vi "Environment Step Type - Configure.vi"(9 "Value Expression In":string, 10 "Environment Setting":T1, 11 "Sequence Context In":refnum<k7>) -> (0 "error out":errorcluster, 1 "Setting name":string, 2 "Value Expression Out":string, 3 "Setting out":T1)   [LabVIEW 2013]
uses:
  <instrlib>/Driver Simulation/Fixture/EnvironmentSettings.ctl
  <vilib>/addons/TestStand/_TSUtility.llb/TestStand - Start Modal Dialog (Sequence Context).vi
  <vilib>/addons/TestStand/_TSUtility.llb/TestStand - End Modal Dialog (Sequence Context).vi
  <instrlib>/Driver Simulation/Fixture.lvlib
panel:
  in  "Cancel":bool
  in  "Value":refnum<k7>(container)
  in  "OK":bool
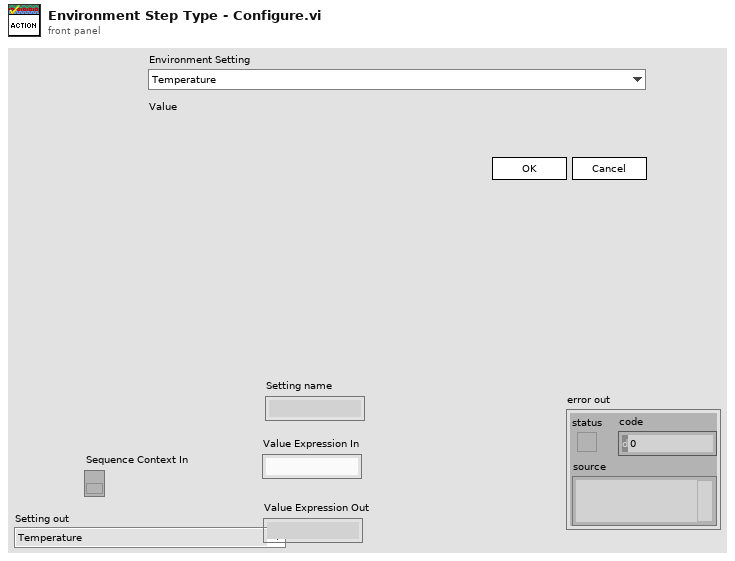
[diagram p1: front panel]
types:
  T1 = typedef "Driver Simulation.lvlib/Fixture.lvlib/EnvironmentSettings.ctl" = enum16{"Temperature", "Light Intensity"}
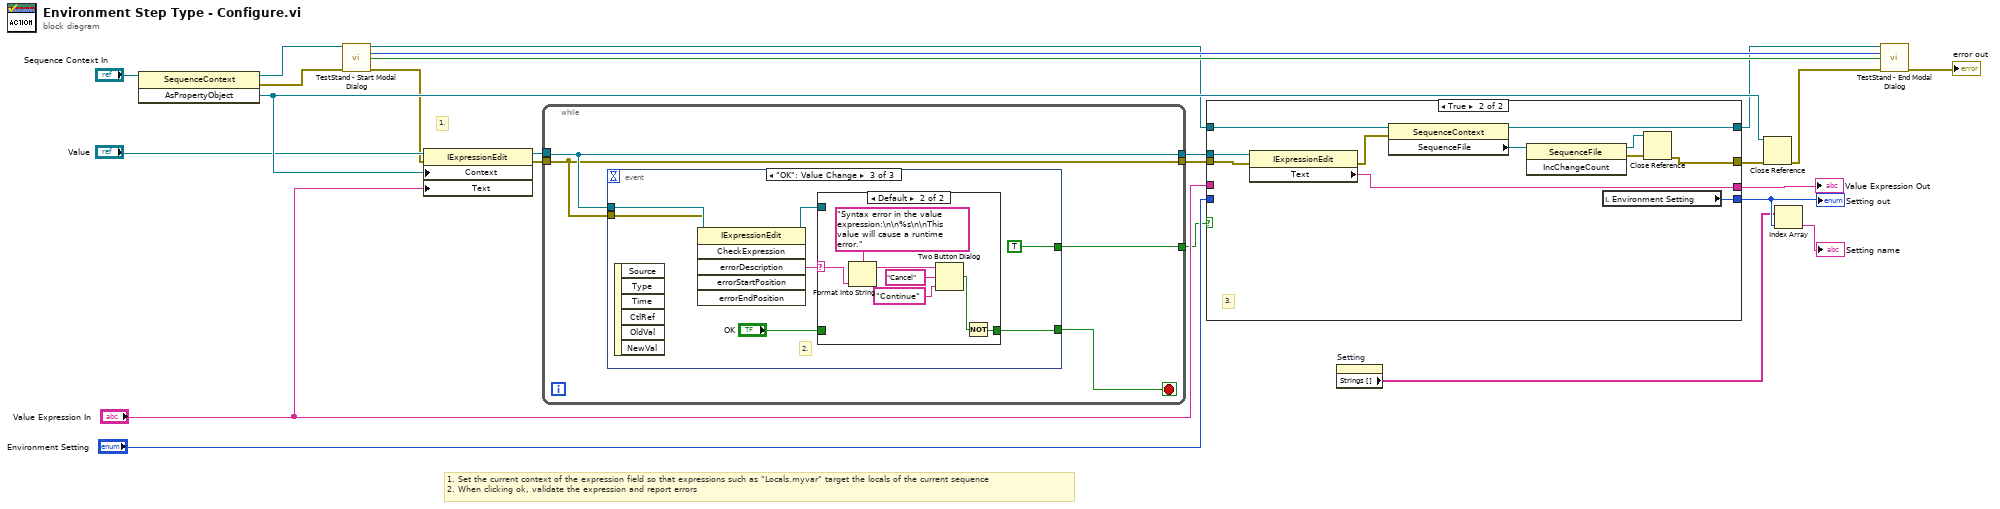
[diagram p0: block diagram]
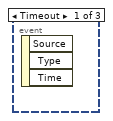
[diagram p3: hidden frame]
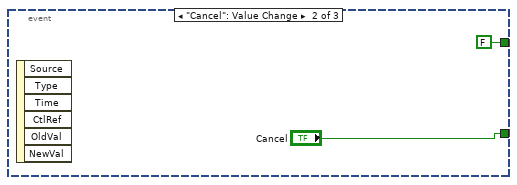
[diagram p4: hidden frame]
diagram:
  # "1. Set the current context of the expression field so that expressions such as \"Locals.myvar\" target the locals of the current sequence\n2. When clicking ok, validate the expression and report errors"
  # "1."
  n1 = invoke class="SequenceContext" method="AsPropertyObject"(reference="Sequence Context In") -> (reference out=w9:refnum<k7>, error out=w3:errorcluster, "AsPropertyObject"=w21:refnum<k7>)  [unwired: 2 in]
  n2 = call-poly <vilib>:"TestStand - Start Modal Dialog.vi"("Sequence Context In"=w9, "error in (no error)"=w3) -> ("Sequence Context Out"=w2:refnum<k7>, "Modal ID"=w5:i32, "VI Originally Open"=w4:bool, "error out"=w8:errorcluster)  [unwired: 9 in, 1 out]
  n3 = property class="IExpressionEdit"(reference="Value", error in=w8, "Context"=w21, "Text"="Value Expression In") -> (reference out=w23:refnum<k7>, error out=w22:errorcluster)
  n4 = while {
    tunnel: w23 -> [w27]
    tunnel: w22 -> [w26]
    tunnel: [w26] -> w19
    tunnel: [w27] -> w16
    tunnel: [w28] -> w10
    stop <- w25 stop-if-true
    n5 = event shown="[2] \"OK\": Value Change" {
      selector: _ -> [_ _ _]
      dyn-events: _ -> [_ _ _]
      timeout: _ -> [_ _ _]
      tunnel: [_ FALSE ("OK") TRUE ("OK")] -> w28
      tunnel: w27 -> [_ _ w36]
      tunnel: w26 -> [_ _ w35]
      tunnel: [_ "Cancel" w34] -> w25
      event Timeout {
        n6 = event-data() -> ()  [unwired: 1 in, 3 out]
      }
      event "Cancel": Value Change {
        n7 = event-data() -> ()  [unwired: 1 in, 6 out]
      }
      event "OK": Value Change {
        # "2."
        n8 = event-data() -> ()  [unwired: 1 in, 6 out]
        n9 = invoke class="IExpressionEdit" method="CheckExpression"(reference=w36, error in=w35) -> (reference out=w31:refnum<k7>, "errorDescription"=w32:string)  [unwired: 4 in, 4 out]
        n10 = case shown="Default" w32 {
          selector: w32 -> [_ w45]
          tunnel: [w38 w40] -> w34
          tunnel: "OK" -> [w38 _]
          tunnel: w31 -> [_ _]
          frame "" {
          }
          frame Default {
            n11 = Format Into String(format string="Syntax error in the value expression:\n\n%s\n\nThis value will cause a runtime error.", w45) -> (resulting string=w43:string)  [unwired: 2 in, 1 out]
            n12 = Two Button Dialog(message=w43, 1:"Continue" ("T button name (\"OK\")"), 2:"Cancel" ("T button name (\"OK\")")) -> (T button?=w39:bool)
            n13 = Not(x=w39) -> (.not. x?=w40:bool)
          }
        }
      }
    }
  }
  n14 = case shown="True" w10 {
    tunnel: w19 -> [w47 w60]
    tunnel: [w49 w59] -> w18
    tunnel: [w47 w51] -> w17
    tunnel: w16 -> [_ w58]
    tunnel: [w48 w57] -> w13
    tunnel: "Value Expression In" -> [w49 _]
    tunnel: "Environment Setting" -> [w48 _]
    tunnel: w2 -> [w46 w54]
    tunnel: [w46 w50] -> w1
    frame False {
    }
    frame True {
      # "3."
      n15 = property class="IExpressionEdit"(reference=w58, error in=w60) -> (error out=w55:errorcluster, "Text"=w59:string)  [unwired: 1 out]
      n16 = property class="SequenceContext"(reference=w54, error in=w55) -> (reference out=w50:refnum<k7>, "SequenceFile"=w56:refnum<k7>)  [unwired: 1 out]
      n17 = invoke class="SequenceFile" method="IncChangeCount"(reference=w56) -> (reference out=w52:refnum<k7>, error out=w53:errorcluster)  [unwired: 2 in, 1 out]
      n18 = local read "Environment Setting"() -> (w57:T1)
      n19 = Close Reference(reference=w52, error in (no error)=w53) -> (error out=w51:errorcluster)
    }
  }
  "Value Expression Out" <- w18
  "Setting out" <- w13
  n20 = property on="Setting" class="Enum (strict)"() -> ("Strings []"=w12:string[])  [unwired: 2 in, 2 out]
  n21 = Close Reference(reference=w21, error in (no error)=w17) -> (error out=w7:errorcluster)
  n22 = Index Array(array=w12, index=w13) -> (element=→"Setting name":string)
  n23 = call-poly <vilib>:"TestStand - End Modal Dialog.vi"("Sequence Context In"=w1, "Modal ID"=w5, "VI Originally Open"=w4, "error in (no error)"=w7) -> ("error out"=→"error out":errorcluster)  [unwired: 11 in]
